vi "Start.vi"(8 "error in (no error)":errorcluster, 10 "Message in":refnum<class "StartMessage.lvclass">, 11 "RSA in":refnum<class "RSA.lvclass">) -> (0 "error out":errorcluster, 3 "RSA out":refnum<class "RSA.lvclass">)   [LabVIEW 2012, in "RSA.lvclass"]
doc: "This member function is called when the statemachine in the run.vi receives an 'start' command. It relays the message to all observers of the component.\n\nOverride this member function in your derived class if you need additional start functionality (but don't forget to call the parent method)."
uses:
  RSA.lvclass
  <vilib>/Distrio/Murmex/StartMessage/StartMessage.lvclass
  <vilib>/Distrio/Murmex/Murmex/Murmex.lvclass
  <vilib>/Distrio/Murmex/ProceedMessage/ProceedMessage.lvclass
  RSA.lvclass/RSA.ctl
panel:
  # "This member function is called when the statemachine in the run.vi receives an 'start' command. It relays the message to all observers of the component.\n\nOverride this member function in your derived class if you need additional start functionality (but don't forget to call the parent method)."
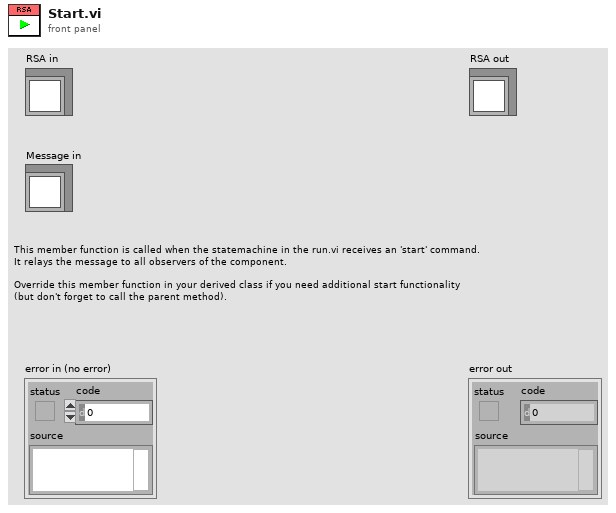
[diagram p1: front panel]
types:
  T1 = typedef "RSA.lvclass/starting shape.ctl" = enum16{"Load shape", "Midrange"}
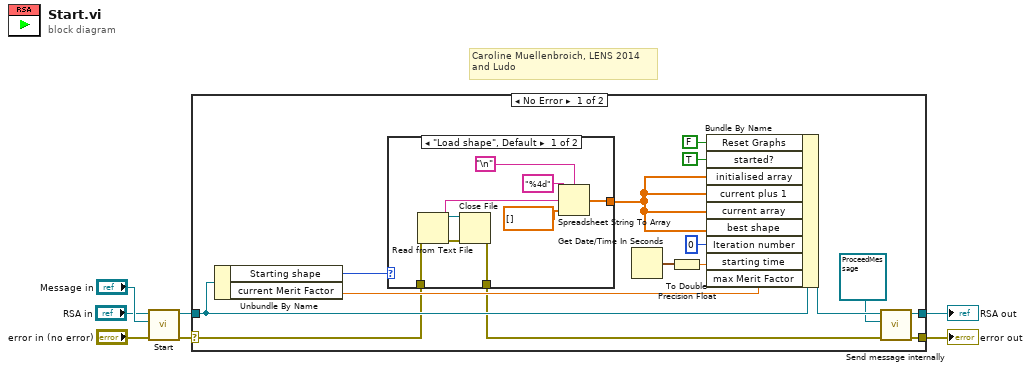
[diagram p0: block diagram]
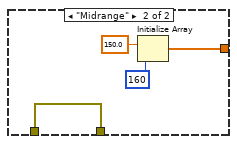
[diagram p2: hidden frame]
diagram:
  # "Caroline Muellenbroich, LENS 2014\nand Ludo"
  n1 = call-parent "Start.vi"("error in (no error)"="error in (no error)", "Message in"="Message in", "Murmex in"="RSA in") -> ("error out"=w4:errorcluster, "Murmex out"=w3:refnum<class "RSA.lvclass">)  [unwired: 7 in]
  n2 = case shown="No Error" w4 {
    selector: w4 -> [w11 w36]
    tunnel: w3 -> [w22 w37]
    tunnel: [w18 w37] -> w2
    tunnel: [w19 w36] -> w1
    frame No Error {
      n3 = Unbundle By Name(w22) -> ("Starting shape"=w13:T1, "current Merit Factor"=w14:dbl)
      n4 = case shown="\"Load shape\", Default" w13 {
        tunnel: [w27 w33] -> w12
        tunnel: w11 -> [w26 w32]
        tunnel: [w24 w32] -> w10
        frame "Load shape", Default {
          n5 = Read from Text File(error in=w26) -> (refnum out=w29:refnum<file>, text=w31:string, error out=w25:errorcluster)  [unwired: 1 in, 3 out]
          n6 = Close File(refnum=w29, error in=w25) -> (error out=w24:errorcluster)  [unwired: 1 out]
          n7 = Spreadsheet String To Array(delimiter (Tab)="\n", format string="%4d", spreadsheet string=w31, array type (2D Dbl)=dbl[] [] ("run time Cluster.1x160  Voltage Map")) -> (array=w27:dbl[])
        }
        frame "Midrange" {
          n8 = Initialize Array(150.0 ("element"), 160 ("dimension size")) -> (w33:dbl[])
        }
      }
      n9 = Get Date/Time In Seconds() -> (seconds since 1Jan1904=w21:timestamp)
      n10 = To Double Precision Float(number=w21) -> (double precision float=w20:dbl)
      n11 = Bundle By Name(cluster=w22, "Reset Graphs"=FALSE ("Run time cluster.Reset Graphs"), "started?"=TRUE ("Run time cluster.started?"), "initialised array"=w12, "current plus 1"=w12, "current array"=w12, "best shape"=w12, "Iteration number"=0 ("Run time cluster.Iteration number"), "starting time"=w20, "max Merit Factor"=w14) -> (w17:refnum<class "RSA.lvclass">)
      n12 = call <vilib>:"Send message internally.vi"("error in (no error)"=w10, "Message"=refnum<class "ProceedMessage.lvclass"> refnum ("ProceedMessage"), "Murmex in"=w17) -> ("error out"=w19:errorcluster, "Murmex out"=w18:refnum<class "RSA.lvclass">)  [unwired: 7 in]
    }
    frame Error {
    }
  }
  "error out" <- w1
  "RSA out" <- w2
